vi "Read Shifter from File.vi"(8 "error in (no error)":errorcluster, 10 "XML File Path":path, 11 "Shifter in":refnum<class "Shifter.lvclass">) -> (0 "error out":errorcluster, 3 "Shifter out":refnum<class "Shifter.lvclass">)   [LabVIEW 2013]
uses:
  Shifter.lvclass
  <vilib>/Utility/xml.llb/Read From XML File(string).vi
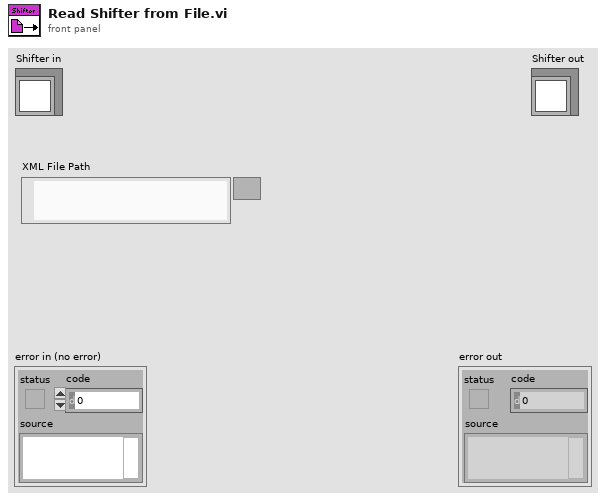
[diagram p1: front panel]
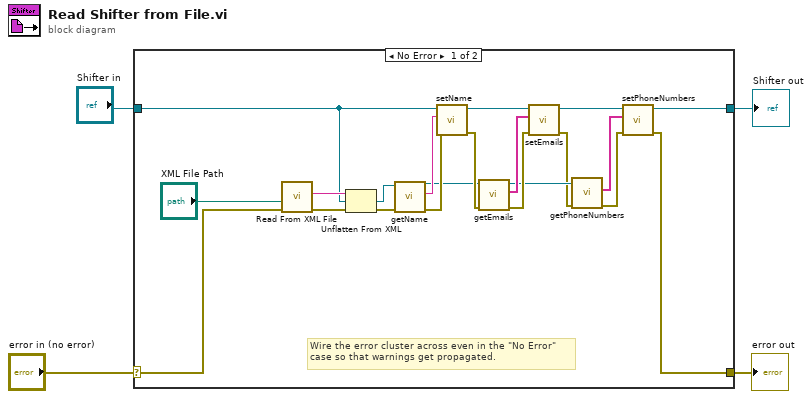
[diagram p0: block diagram]
diagram:
  n1 = case shown="No Error" "error in (no error)" {
    selector: "error in (no error)" -> [w24 w27]
    tunnel: [w5 w27] -> w3
    tunnel: [w6 w26] -> w1
    tunnel: "Shifter in" -> [w19 w26]
    frame No Error {
      # "Wire the error cluster across even in the \"No Error\"\ncase so that warnings get propagated."
      n2 = call-poly <vilib>:"Read From XML File.vi"("error in (no error)"=w24, "XML File Path"="XML File Path") -> ("error out"=w23:errorcluster, "XML Elements"=w22:string)  [unwired: 7 in, 1 out]
      n3 = Unflatten From XML(xml string=w22, type=w19, error in (no error)=w23) -> (value=w20:refnum<class "Shifter.lvclass">, error out=w21:errorcluster)
      n4 = call-dynamic "getName.vi"("error in (no error)"=w21, "Shifter in"=w20) -> ("error out"=w17:errorcluster, "name"=w18:string, "Shifter out"=w15:refnum<class "Shifter.lvclass">)  [unwired: 7 in]
      n5 = call-dynamic "setName.vi"("error in (no error)"=w17, "name"=w18, "Shifter in"=w19) -> ("error out"=w16:errorcluster, "Shifter out"=w10:refnum<class "Shifter.lvclass">)  [unwired: 7 in]
      n6 = call-dynamic "getEmails.vi"("error in (no error)"=w16, "Shifter in"=w15) -> ("error out"=w14:errorcluster, "emails"=w13:string[], "Shifter out"=w12:refnum<class "Shifter.lvclass">)  [unwired: 7 in]
      n7 = call-dynamic "setEmails.vi"("error in (no error)"=w14, "emails"=w13, "Shifter in"=w10) -> ("error out"=w11:errorcluster, "Shifter out"=w9:refnum<class "Shifter.lvclass">)  [unwired: 7 in]
      n8 = call-dynamic "getPhoneNumbers.vi"("error in (no error)"=w11, "Shifter in"=w12) -> ("error out"=w8:errorcluster, "phoneNumbers"=w7:string[])  [unwired: 7 in, 1 out]
      n9 = call-dynamic "setPhoneNumbers.vi"("error in (no error)"=w8, "phoneNumbers"=w7, "Shifter in"=w9) -> ("error out"=w5:errorcluster, "Shifter out"=w6:refnum<class "Shifter.lvclass">)  [unwired: 7 in]
    }
    frame Error {
    }
  }
  "error out" <- w3
  "Shifter out" <- w1
